vi "DHT22_photo_force.vi"() -> ()   [LabVIEW 2013]
uses:
  <vilib>/Instr/_visa.llb/VISA Configure Serial Port (Instr).vi
  <vilib>/Utility/file.llb/Write To Spreadsheet File (string).vi
panel:
  out "Pressure":dbl[](graph)
  out "Pressure (a.u.)":dbl
  out "read buffer":string
  out "Light Sensor":dbl[](graph)
  out "Light Intensity (a.u.)":dbl
  out "Temp":dbl[](graph)
  out "Temp (C)":dbl
  out "Humidity":dbl[](graph)
  out "Humidity (%)":dbl
  in  "stop":bool
  # "Arduino Temp, Humidity, Light, Force Sensing"
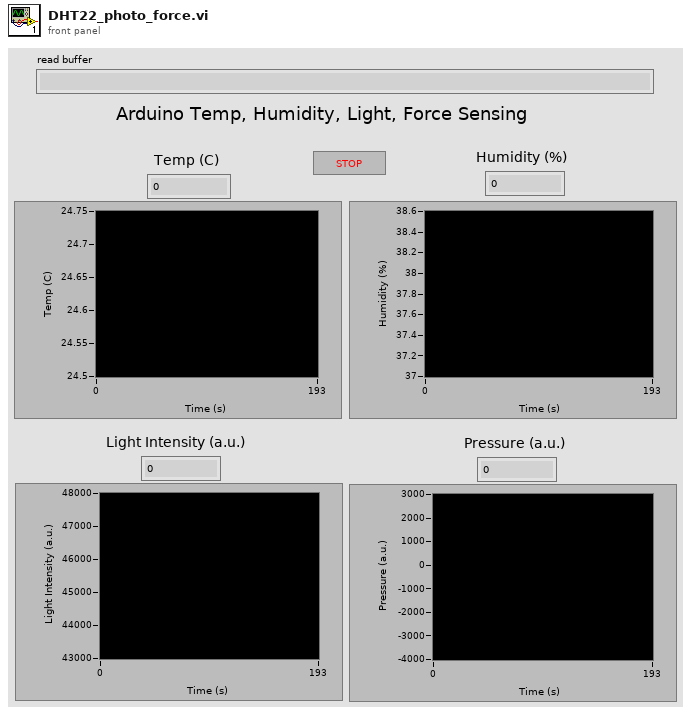
[diagram p1: front panel]
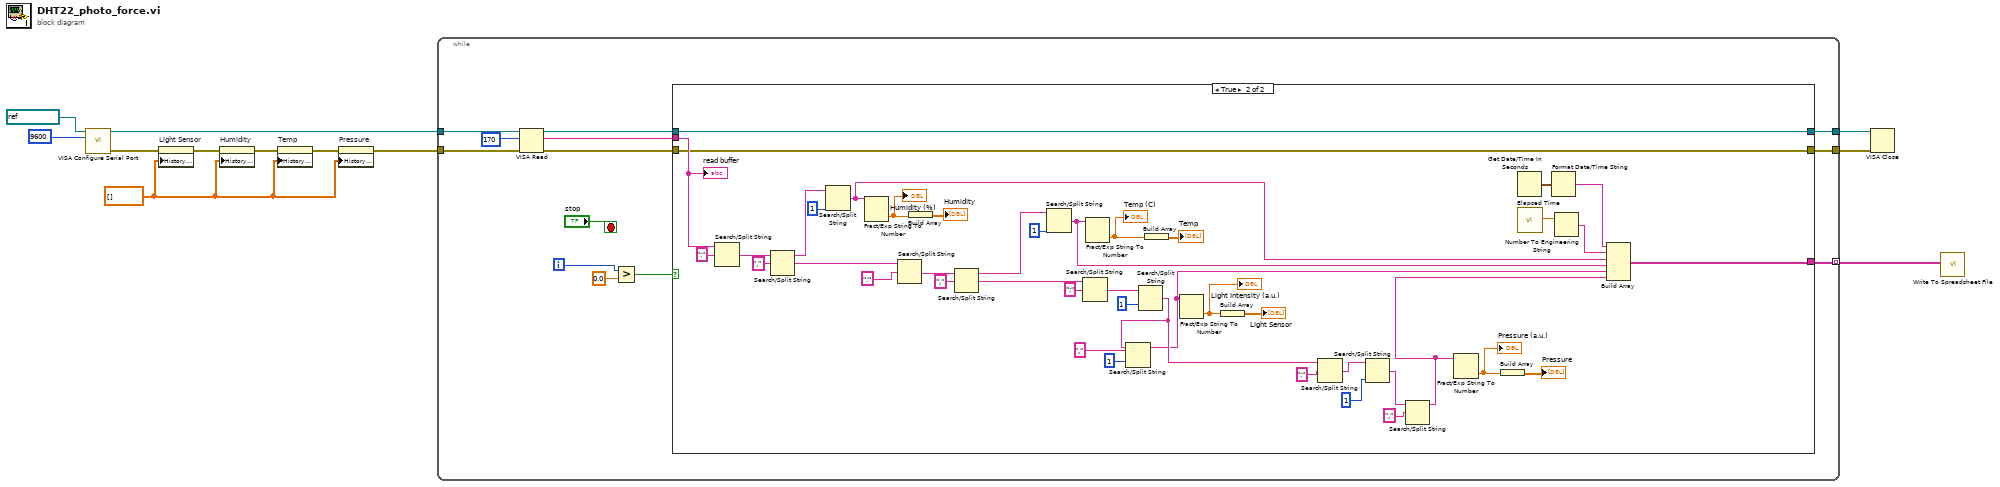
[diagram p0: block diagram]
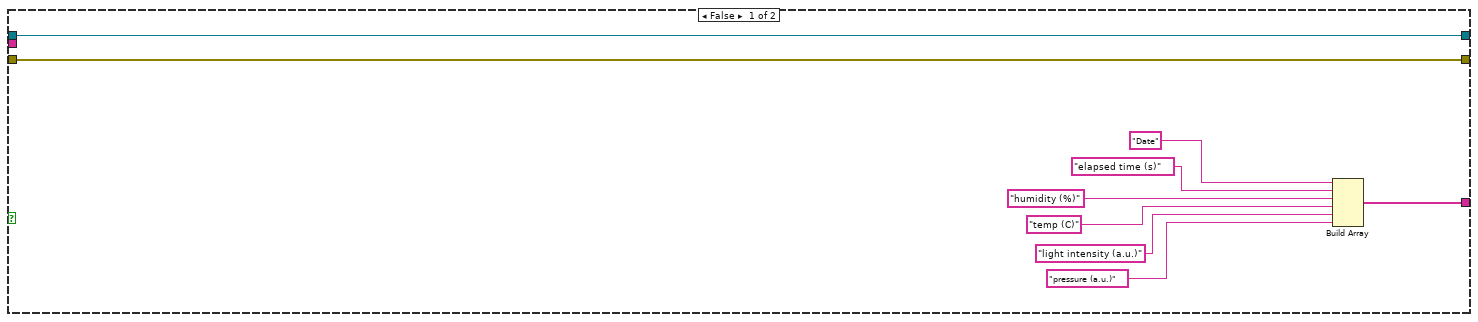
[diagram p2: hidden frame]
diagram:
  w2 = dbl[] [] ("History Data")
  n1 = call-poly "VISA Configure Serial Port"("VISA resource name"=refnum<visa-resource-name> "COM12", "baud rate (9600)"=u32 9600) -> ("VISA resource name out"=w10:refnum<visa-resource-name>, "error out"=w5:errorcluster)  [unwired: 12 in]
  n2 = property on="Light Sensor" class="WFChart (strict)"(error in=w5, "History Data"=w2) -> (error out=w6:errorcluster)  [unwired: 1 in, 1 out]
  n3 = property on="Humidity" class="WFChart (strict)"(error in=w6, "History Data"=w2) -> (error out=w7:errorcluster)  [unwired: 1 in, 1 out]
  n4 = property on="Temp" class="WFChart (strict)"(error in=w7, "History Data"=w2) -> (error out=w4:errorcluster)  [unwired: 1 in, 1 out]
  n5 = property on="Pressure" class="WFChart (strict)"(error in=w4, "History Data"=w2) -> (error out=w3:errorcluster)  [unwired: 1 in, 1 out]
  n6 = while {
    tunnel: w10 -> [w23]
    tunnel: w3 -> [w22]
    tunnel: [w19] -> w12
    tunnel: [w18] -> w11
    tunnel: [w13] -> w1 mode=indexing
    i -> [w16]
    stop <- "stop" stop-if-true
    n7 = VISA Read(VISA resource name=w23, byte count=u32 170, error in (no error)=w22) -> (VISA resource name out=w20:refnum<visa-resource-name>, read buffer=w21:string, error out=w14:errorcluster)  [unwired: 1 out]
    n8 = Greater?(x=w16, y=0.0) -> (0:w15:bool)
    n9 = case shown="True" w15 {
      tunnel: w21 -> [_ w77]
      tunnel: w20 -> [w34 w58]
      tunnel: w14 -> [w33 w57]
      tunnel: [w34 w58] -> w19
      tunnel: [w33 w57] -> w18
      tunnel: [w26 w50] -> w13
      frame False {
        n10 = Build Array("Date" ("element"), "elapsed time (s)", "humidity (%)", "temp (C)", "light intensity (a.u.)", "pressure (a.u.)") -> (w26:string[])
      }
      frame True {
        n11 = Search/Split String(string=w77, search string/char (-)=":") -> (match + rest of string=w74:string)  [unwired: 1 in, 2 out]
        n12 = Search/Split String(string=w74, search string/char (-)=",") -> (substring before match=w69:string, match + rest of string=w73:string)  [unwired: 1 in, 1 out]
        n13 = Search/Split String(string=w69, offset (0)=1) -> (match + rest of string=w45:string)  [unwired: 1 in, 2 out]
        n14 = Fract/Exp String To Number(string=w45) -> (number=w46:dbl)  [unwired: 3 in, 1 out]
        "Humidity (%)" <- w46
        n15 = Search/Split String(string=w73, search string/char (-)=":") -> (match + rest of string=w70:string)  [unwired: 1 in, 2 out]
        n16 = Build Array(w46) -> (→"Humidity":dbl[])
        n17 = Search/Split String(string=w70, search string/char (-)=",") -> (substring before match=w65:string, match + rest of string=w61:string)  [unwired: 1 in, 1 out]
        n18 = Search/Split String(string=w65, offset (0)=1) -> (match + rest of string=w42:string)  [unwired: 1 in, 2 out]
        n19 = Search/Split String(string=w61, search string/char (-)=":") -> (match + rest of string=w59:string)  [unwired: 1 in, 2 out]
        n20 = Fract/Exp String To Number(string=w42) -> (number=w52:dbl)  [unwired: 3 in, 1 out]
        "Temp (C)" <- w52
        n21 = Search/Split String(string=w59, offset (0)=1) -> (match + rest of string=w39:string)  [unwired: 1 in, 2 out]
        n22 = Search/Split String(string=w39, search string/char (-)=",", offset (0)=1) -> (substring before match=w38:string)  [unwired: 2 out]
        n23 = Build Array(w52) -> (→"Temp":dbl[])
        n24 = Fract/Exp String To Number(string=w38) -> (number=w47:dbl)  [unwired: 3 in, 1 out]
        "Light Intensity (a.u.)" <- w47
        n25 = Build Array(w47) -> (→"Light Sensor":dbl[])
        n26 = Search/Split String(string=w39, search string/char (-)=":") -> (match + rest of string=w53:string)  [unwired: 1 in, 2 out]
        n27 = Search/Split String(string=w53, offset (0)=1) -> (match + rest of string=w36:string)  [unwired: 1 in, 2 out]
        n28 = Search/Split String(string=w36, search string/char (-)=",") -> (substring before match=w35:string)  [unwired: 1 in, 2 out]
        n29 = Fract/Exp String To Number(string=w35) -> (number=w48:dbl)  [unwired: 3 in, 1 out]
        "Pressure (a.u.)" <- w48
        n30 = Build Array(w48) -> (→"Pressure":dbl[])
        n31 = Get Date/Time In Seconds() -> (seconds since 1Jan1904=w51:timestamp)
        n32 = call "Elapsed Time"() -> ("Elapsed Time (s)"=w49:dbl)  [unwired: 12 in, 7 out]
        n33 = Format Date/Time String(seconds (now)=w51) -> (date/time string=w44:string)  [unwired: 2 in]
        n34 = Number To Engineering String(4:w49) -> (0:w43:string)  [unwired: 3 in]
        n35 = Build Array(w44, w43, w45, w42, w38, w35) -> (w50:string[])
        "read buffer" <- w77
      }
    }
  }
  n36 = VISA Close(VISA resource name=w12, error in (no error)=w11) -> ()  [unwired: 1 out]
  n37 = call-poly <vilib>:"Write To Spreadsheet File.vi"("2D data"=w1) -> ()  [unwired: 7 in, 1 out]
